vi "ELVIS III v1.0 AI Global.vi"() -> ()   [LabVIEW 2021]
panel:
  in  "AI 1 Sample Default Channel CNT":u8=12
  in  "AI 1 Sample Default Ticks":u32=1000
  in  "AI 1 Sample Bank Default Config":u8[](array[numeric])=[8, 9, 10, 11, 12, 13, 14, 15, 0, 1, 2, 3]
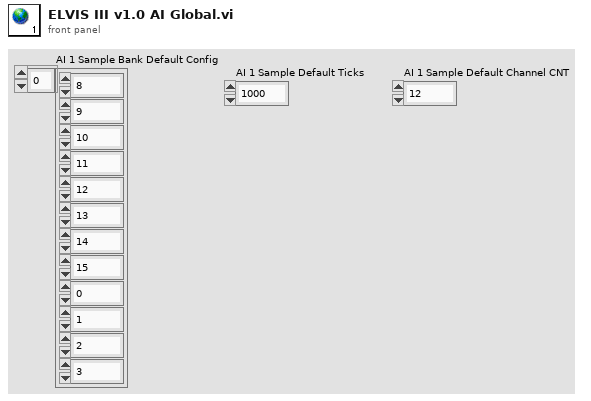
[diagram p1: front panel]
diagram:
